vi "ContDecodeProgramIterations2.vi"(11 "Continuous Program in":string[][](array[string])) -> (3 "Continuous Program out":string[][](array[string]))   [LabVIEW 2018, in "ContinousLoop.lvlib"]
uses:
  ContinousLoop.lvlib
  Config/Config.lvlib
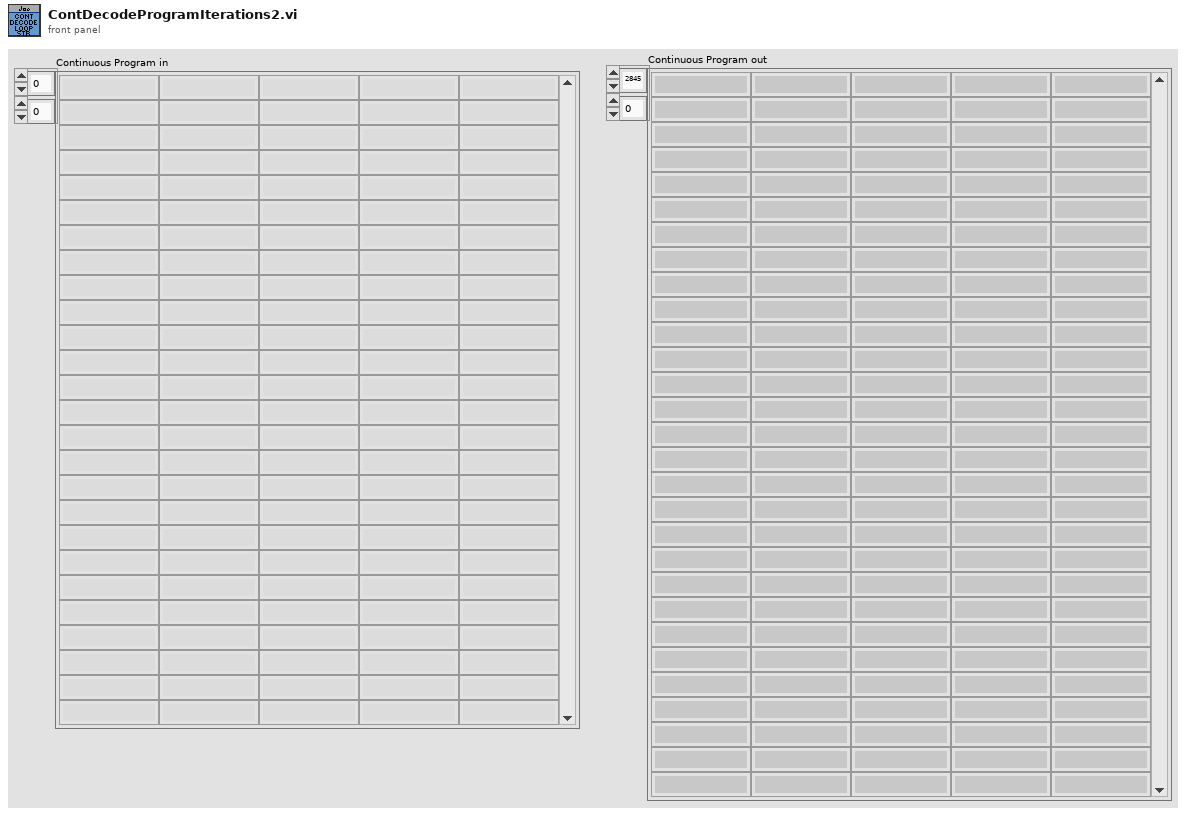
[diagram p1: front panel]
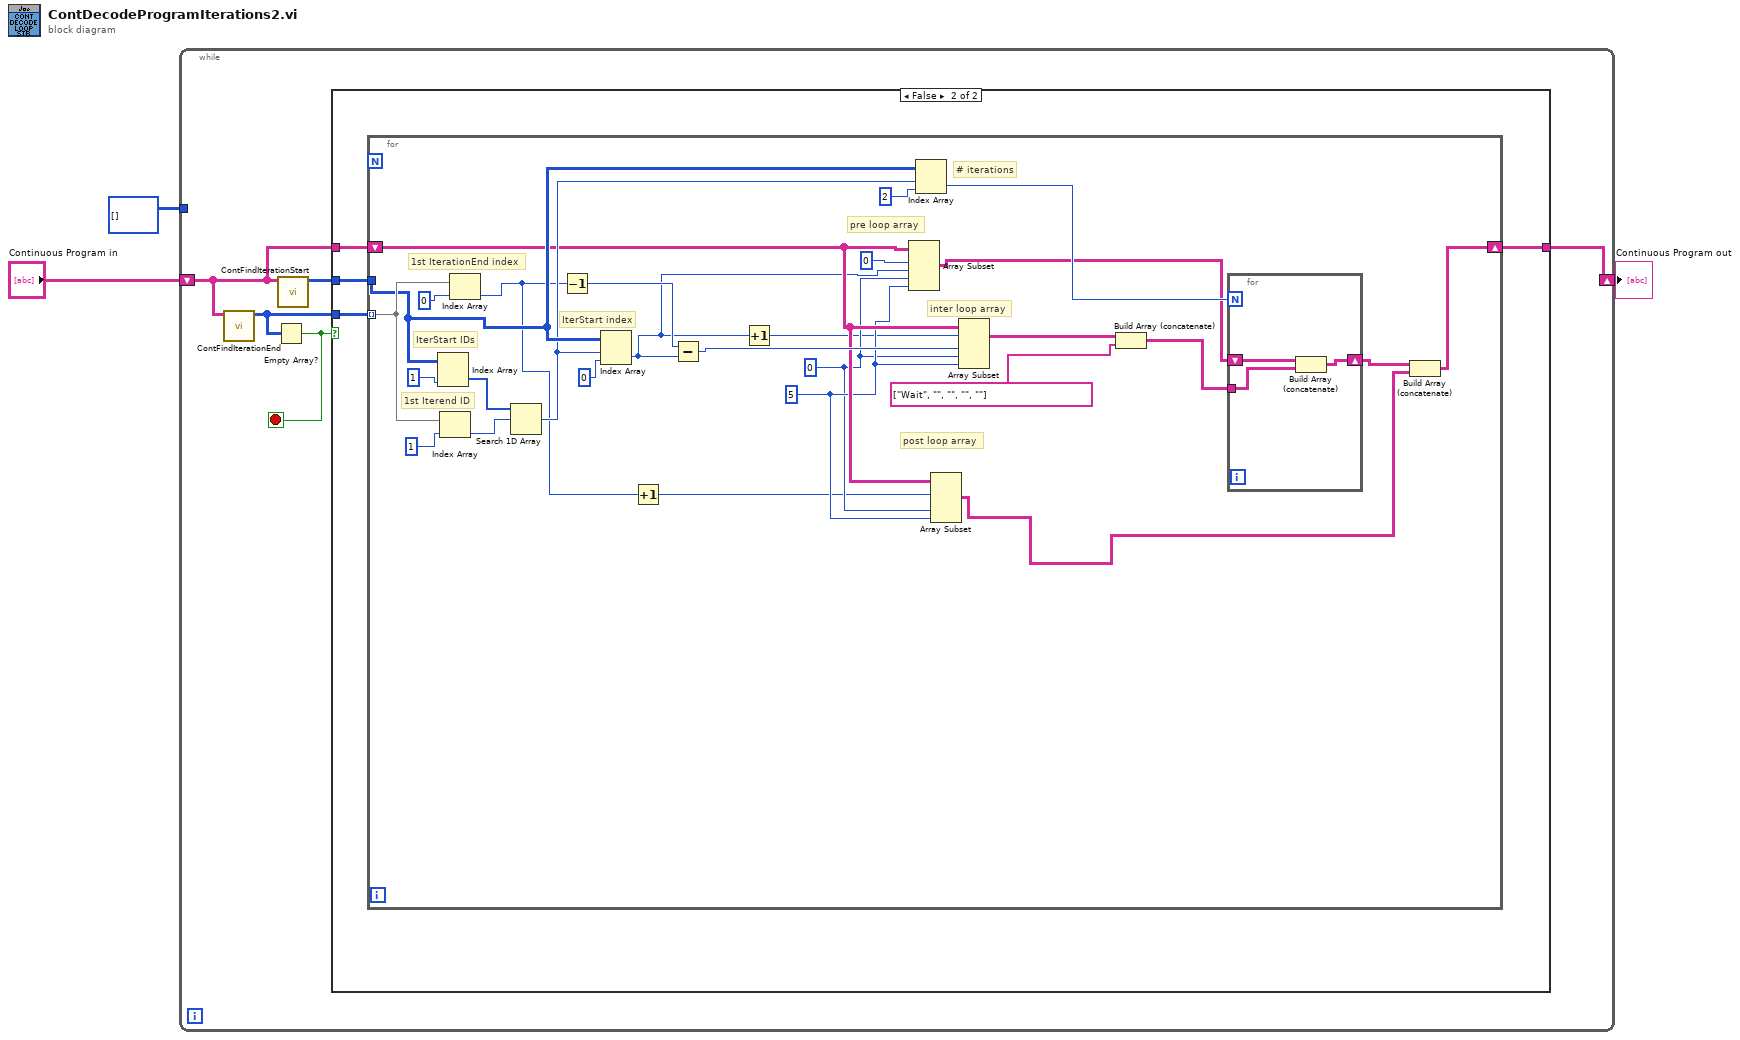
[diagram p0: block diagram]
diagram:
  n1 = while {
    tunnel: i32[][] [] -> [_]
    shift-right: [w8] -> w3
    shift-left: "Continuous Program in" -> [w4]
    stop <- w6 stop-if-true
    n2 = call "ContFindIterationEnd.vi"("Continuous Program in"=w4) -> ("Array out"=w7:i32[][])  [unwired: 10 in]
    n3 = Empty Array?(array=w7) -> (empty?=w6:bool)
    n4 = call "ContFindIterationStart.vi"("ItemNames"=w4) -> ("Array"=w5:i32[][])  [unwired: 10 in]
    n5 = case shown="False" w6 {
      tunnel: w5 -> [_ w13]
      tunnel: w4 -> [w9 w12]
      tunnel: [w9 w11] -> w8
      tunnel: w7 -> [_ w10]
      frame True {
      }
      frame False {
        n6 = for {
          tunnel: w13 -> [w31]
          tunnel: w10 -> [w39] mode=indexing
          shift-right: [w15] -> w11
          shift-left: w12 -> [w24]
          w23 = 5 ("length")
          w22 = 0 ("index")
          # "IterStart index"
          # "IterStart IDs"
          # "1st Iterend ID"
          # "1st IterationEnd index"
          # "# iterations"
          # "inter loop array"
          # "pre loop array"
          # "post loop array"
          n7 = Index Array(array=w31, index (col)=1 ("index")) -> (element=w37:i32[])  [unwired: 1 in]
          n8 = Index Array(array=w39, index=1 ("disabled index (col)")) -> (element=w35:i32)
          n9 = Index Array(array=w39, index=0 ("disabled index (col)")) -> (element=w19:i32)
          n10 = Search 1D Array(1D array=w37, element=w35) -> (index of element=w29:i32)  [unwired: 1 in]
          n11 = Decrement(x=w19) -> (x-1=w27:i32)
          n12 = Index Array(array=w31, index (row)=w29, index (col)=0 ("index")) -> (element=w21:i32)
          n13 = Increment(x=w19) -> (x+1=w18:i32)
          n14 = Subtract(x=w27, y=w21) -> (x-y=w41:i32)
          n15 = Increment(x=w21) -> (x+1=w20:i32)
          n16 = Array Subset(array=w24, index (row)=0 ("length"), length (row)=w21, index (col)=w22, length (col)=w23) -> (w14:string[][])
          n17 = Index Array(array=w31, index (row)=w29, index (col)=2 ("disabled index (col)")) -> (element=w38:i32)
          n18 = Array Subset(array=w24, index (row)=w18, index (col)=w22, length (col)=w23) -> (w16:string[][])  [unwired: 1 in]
          n19 = Array Subset(array=w24, index (row)=w20, length (row)=w41, index (col)=w22, length (col)=w23) -> (w40:string[][])
          n20 = Build Array (concatenate)(w40, string[] ["Wait", "", "", "", ""]) -> (w26:string[][])
          n21 = for {
            N: w38 -> [_]
            tunnel: w26 -> [w42]
            shift-right: [w43] -> w17
            shift-left: w14 -> [w44]
            n22 = Build Array (concatenate)(w44, w42) -> (w43:string[][])
          }
          n23 = Build Array (concatenate)(w17, w16) -> (w15:string[][])
        }
      }
    }
  }
  "Continuous Program out" <- w3
